vi "Write User Tag.vi"(8 "error in":errorcluster, 10 "Label":string, 11 "MB_TCP session in":refnum<class "MB_Master_TCP.lvclass">) -> (0 "error out":errorcluster, 3 "MB session out":refnum<class "MB_Master_TCP.lvclass">)   [LabVIEW 2024, in "Bronkhorst Flexi-Flow ModbusTCP API.lvlib"]
uses:
  Bronkhorst Flexi-Flow ModbusTCP API.lvlib
  <vilib>/Plasmionique/MB Master/MB_Master_TCP/MB_Master_TCP.lvclass
  PDU Address String Params--ring.ctl
  Write String Register.vi
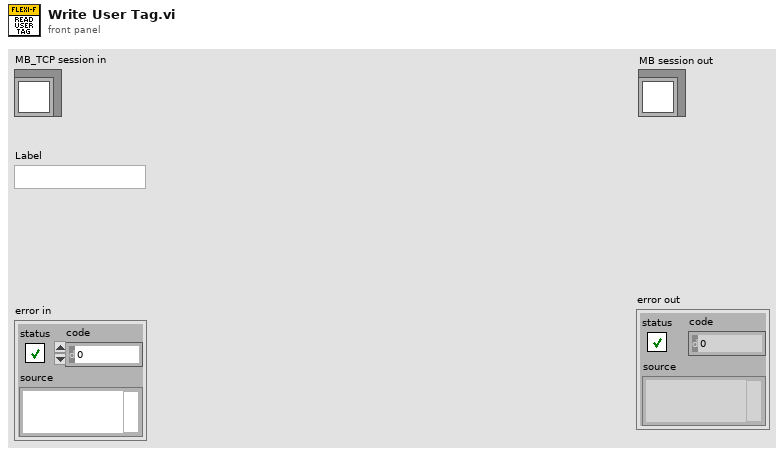
[diagram p1: front panel]
types:
  T1 = typedef "Bronkhorst Flexi-Flow ModbusTCP API.lvlib/PDU Address String Params--ring.ctl" = u16
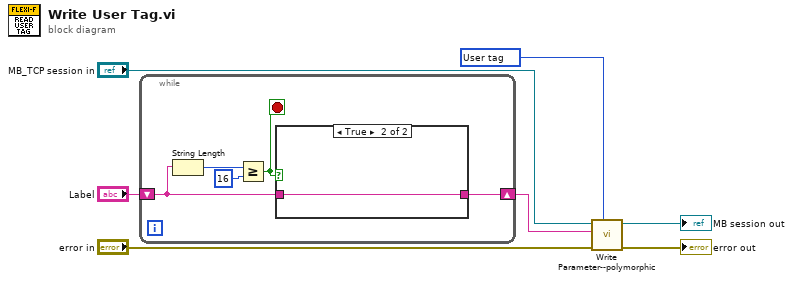
[diagram p0: block diagram]
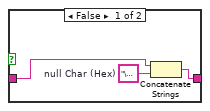
[diagram p2: hidden frame]
diagram:
  w6 = T1 61744 items=["Fluid name"=33160, "Capacity unit"=33272, "User tag"=61744] ("PDU Address String Params")
  n1 = while {
    shift-right: [w10] -> w1
    shift-left: "Label" -> [w9]
    stop <- w8 stop-if-true
    n2 = String Length(string=w9) -> (length=w11:i32)
    n3 = Greater Or Equal?(x=w11, y=16) -> (x >= y?=w8:bool)
    n4 = case shown="True" w8 {
      tunnel: [w13 w16] -> w10
      tunnel: w9 -> [w15 w16]
      frame False {
        w14 = "\u0000"  # null Char (Hex)
        n5 = Concatenate Strings(w15, w14) -> (w13:string)
      }
      frame True {
      }
    }
  }
  n6 = call-poly "Write Parameter--polymorphic.vi"("PDU Address String Params"=w6, "error in"="error in", "String"=w1, "MB_TCP session in"="MB_TCP session in") -> ("error out"=→"error out":errorcluster, "MB session out"=→"MB session out":refnum<class "MB_Master_TCP.lvclass">)  [unwired: 6 in]
